vi "To Variant.vi"(0 "TTLController in":refnum<class "TTLController.lvclass">, 11 "error in (no error)":errorcluster) -> (4 "TTLController out":refnum<class "TTLController.lvclass">, 8 "Array":variant[](array[variant]), 15 "error out":errorcluster)   [LabVIEW 2020, in "TTLController.lvclass"]
uses:
  TTLController.lvclass
  D:/Experiment VIs/Koop/KObject Class/KObject.lvclass
  epl-vi-lib/Koop/KObject Class/KObject.lvclass/KObject.ctl
  TTLController.lvclass/TTLController.ctl
  epl-vi-lib/Koop/KObject Class/Write Version.vi
  epl-vi-lib/Koop/KObject Class/KObject.lvclass
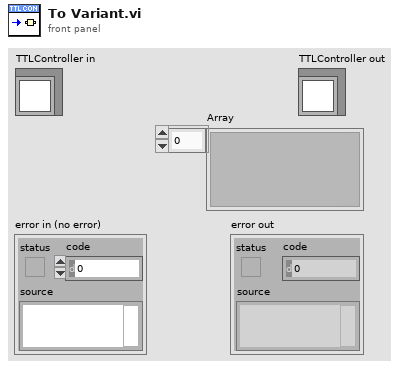
[diagram p1: front panel]
types:
  T1 = typedef "TTLController.lvclass/Serialized.ctl" = cluster{"Name":string, "Start":T2, "Stop":T2, "Pulse":cluster{"Active":bool, "IPI":string, "Width (ms)":dbl}}
  T2 = typedef "TTLController.lvclass/Trigger.ctl" = cluster{"When":string, "Expr":string}
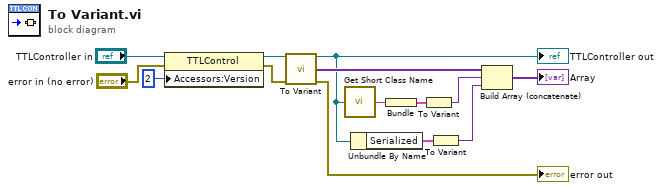
[diagram p0: block diagram]
diagram:
  n1 = property class="TTLControl"(reference="TTLController in", error in="error in (no error)", "Accessors:Version"=2 ("Version")) -> (reference out=w4:refnum<class "TTLController.lvclass">, error out=w3:errorcluster)
  n2 = call-parent "To Variant.vi"("KObject in"=w4, "error in (no error)"=w3) -> ("KObject out"=w5:refnum<class "TTLController.lvclass">, "Array"=w13:variant[], "error out"=→"error out":errorcluster)  [unwired: 11 in]
  "TTLController out" <- w5
  n3 = call "Get Short Class Name.vi"("KObject in"=w5) -> ("Class"=w9:string)  [unwired: 4 in]
  n4 = Unbundle By Name(w5) -> ("Serialized"=w7:T1)
  n5 = Bundle("Class"=w9) -> (w8:cluster{"Class":string})  [unwired: 1 in]
  n6 = To Variant(anything=w8) -> (Variant=w10:variant)
  n7 = To Variant(anything=w7) -> (Variant=w6:variant)
  n8 = Build Array (concatenate)(w13, w10, w6) -> (→"Array":variant[])
